vi "Lavatory_System..vi"(11 "Error_In":errorcluster) -> (15 "Error_Out":errorcluster)   [LabVIEW 2023]
doc: "This is the Main VI that performs the Lavatory system."
uses:
  Controls/Lavatory.ctl
  Controls/Lavatory_Data.ctl
  Controls/Queue_Operation_Select.ctl
  Controls/Timer_Operation_Select.ctl
panel:
  in  "Stop_Simulation":bool
  in  "Alarm_Timer_Limit":dbl=1.0 caption="Alarm Timer Limit" min=1.0 max=300.0
  out "Alarm_Timer_D":dbl caption="Alarm Timer D"
  out "Alarm_Timer_C":dbl caption="Alarm Timer C"
  in  "Lavatory_D_Occupied":bool caption="Lavatory D Occupied"
  in  "Lavatory_C_Occupied":bool caption="Lavatory C Occupied"
  out "Alarm_Timer_B":dbl caption="Alarm Timer B"
  out "Alarm_Timer_A":dbl caption="Alarm Timer A"
  in  "Lavatory_B_Occupied":bool caption="Lavatory B Occupied"
  in  "Lavatory_A_Occupied":bool caption="Lavatory A Occupied"
  out "Rear_Lavatories_Occupied":bool caption="Lavatories\nOccupied"
  out "Front_Lavatories_Occupied":bool caption="Lavatories\nOccupied"
  in  "Alarm_Achnowledge":bool caption="Alarm Achnowledge"
  out "Lavatory":string="Lavatory A,B,C,D"
  out "Alarm":bool
  in  "Seatbelt_Sign_ON":bool caption="Seatbelt Sign ON"
  out "Lavatory_A":T1 caption="Lavatory A"
  out "Lavatory_B":T1 caption="Lavatory B"
  out "Lavatory_D":T1 caption="Lavatory D"
  out "Lavatory_C":T1 caption="Lavatory C"
  # "Airplane Lavatory Signs"
  # "Front"
  # "Rear"
  # "Steward's Area"
  # "Simulation Contols & Indicators"
  # "Secs"
  # "Secs"
  # "Secs"
  # "Secs"
  # "Secs"
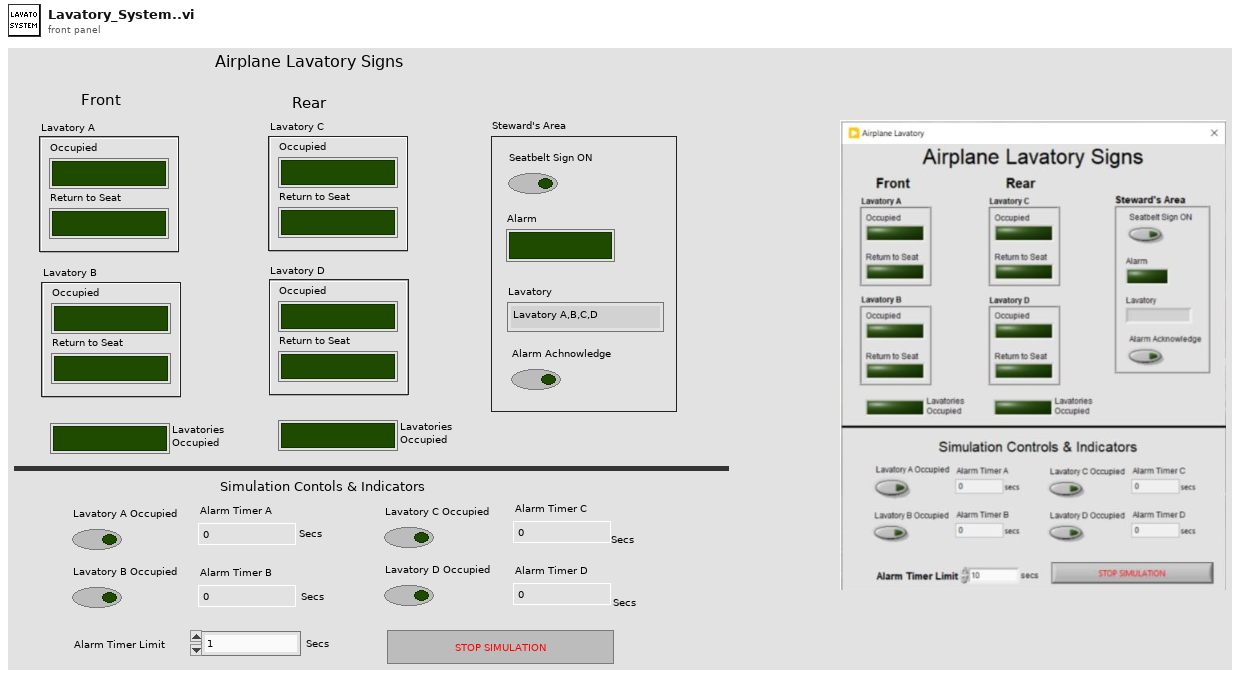
[diagram p1: front panel]
types:
  T1 = typedef "Lavatory.ctl" = cluster{"Occupied":bool, "Return_To_Seat":bool}
  T2 = typedef "Timer_Operation_Select.ctl" = enum16{"Initialize", "Start_Timer", "Time_Out?", "Stop_Timer"}
  T3 = typedef "Queue_Operation_Select.ctl" = enum16{"Obtain_Queue", "Enqueue", "Enqueue_N", "Enqueue_at_End", "Dequeue", "Flush", "Release_Queue"}
  T4 = typedef "Lavatory_Data.ctl" = cluster{"Lavatory":T1, "Rear_Lavatories_Occupied":bool, "Front_Lavatories_Occupied":bool, "Alarm_Time":dbl[], "Alarm":bool, "Alarm_Message":string, "Alarm_Timer_Limit":dbl, "Seatbelt_Sign_ON":bool, "Occupied":bool[], "Return_To_Seat_F":bool[], "Lavatory_Reference":refnum<vi>[], "Time_Out?":bool[], "Lavatory_Controls":refnum<vi>[]}
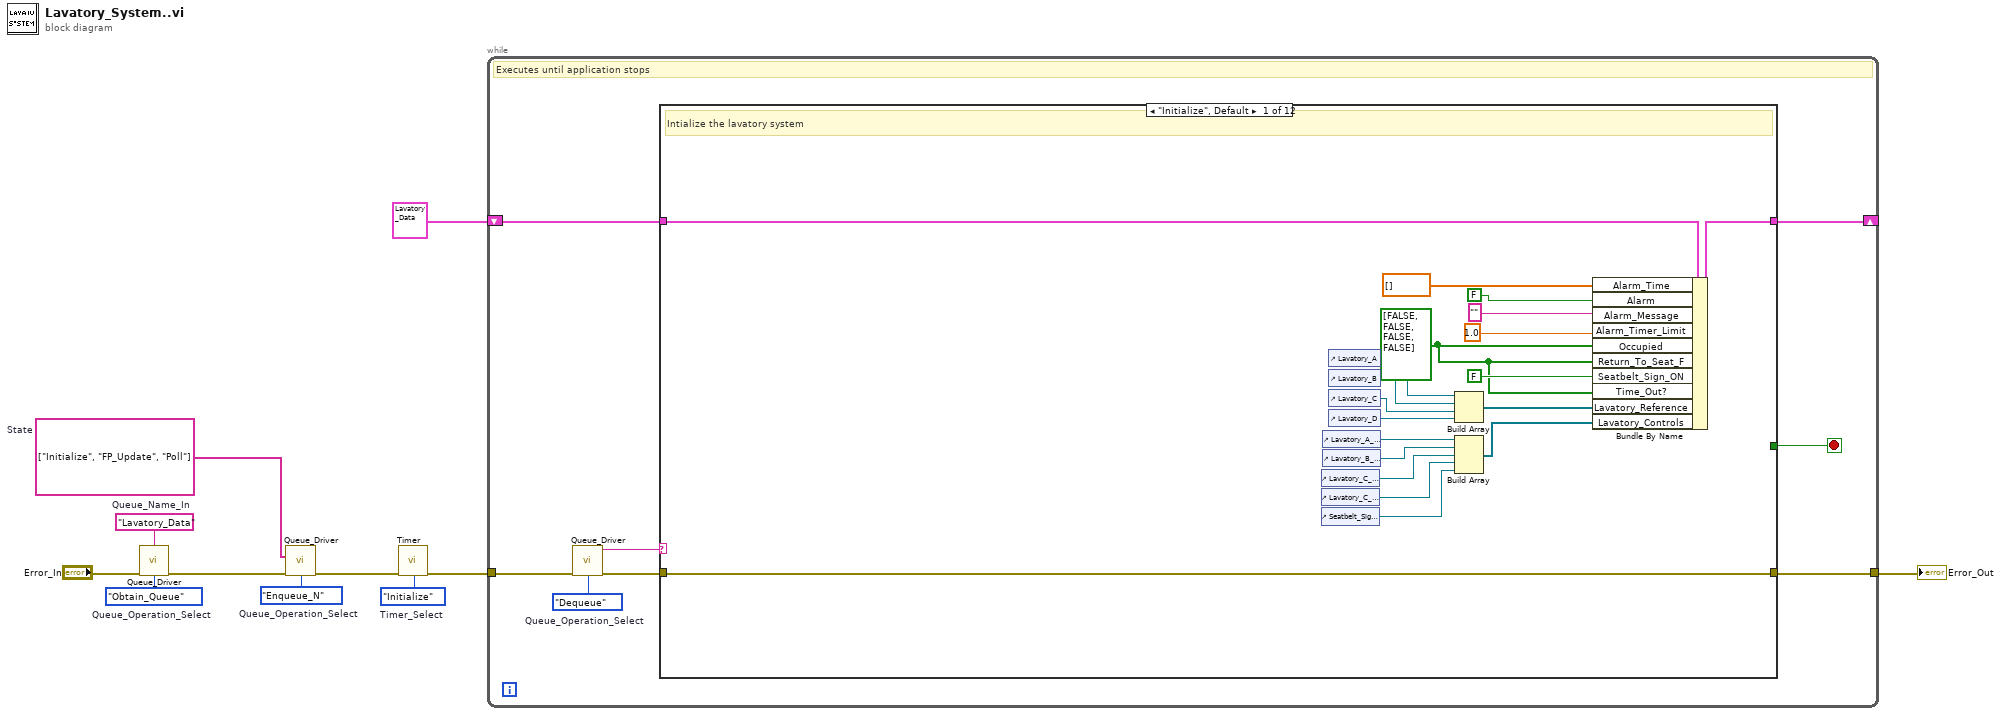
[diagram p0: block diagram]
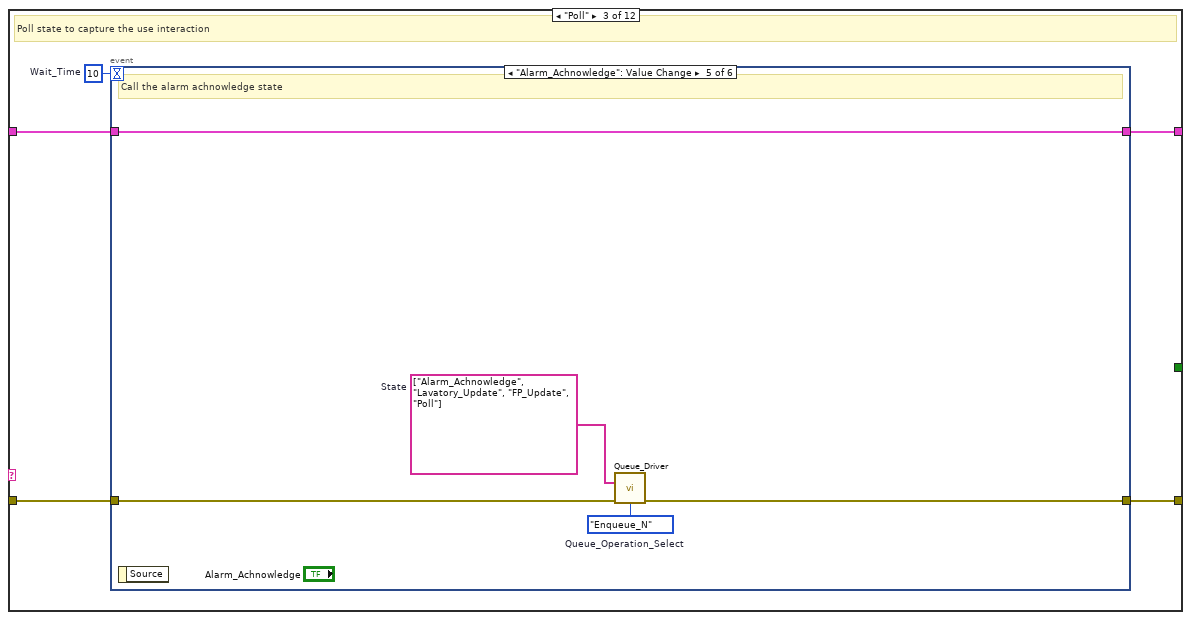
[diagram p3: hidden frame]
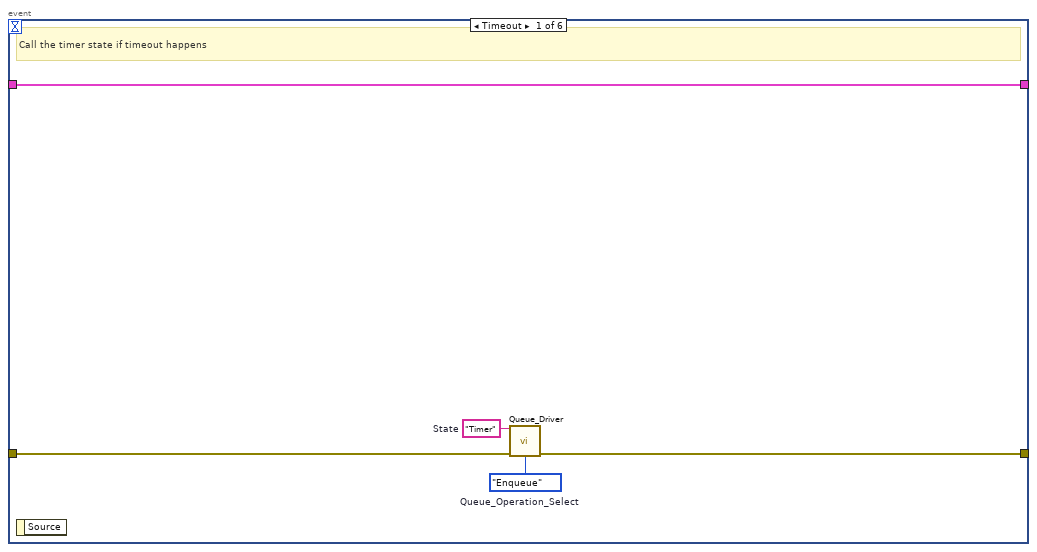
[diagram p4: hidden frame]
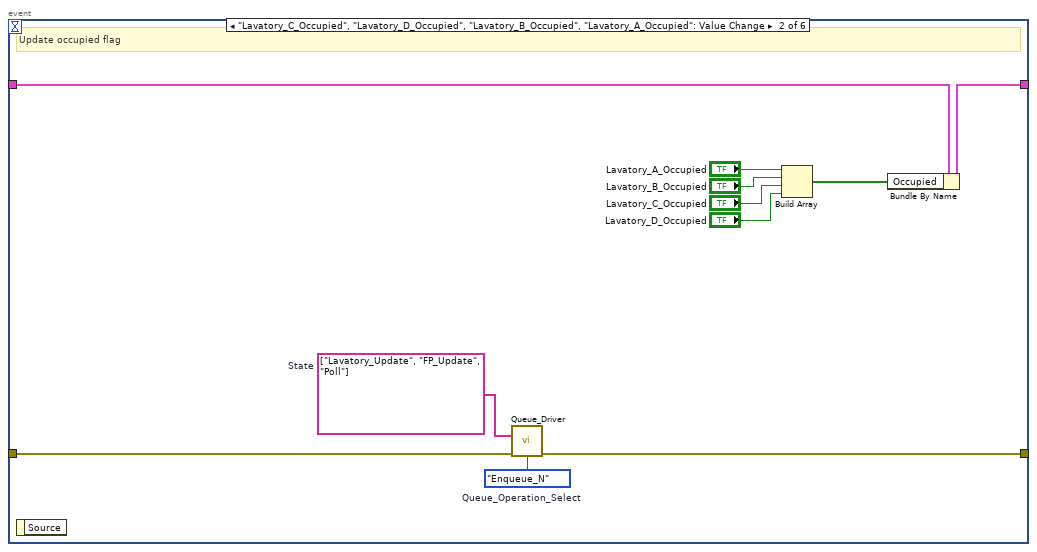
[diagram p5: hidden frame]
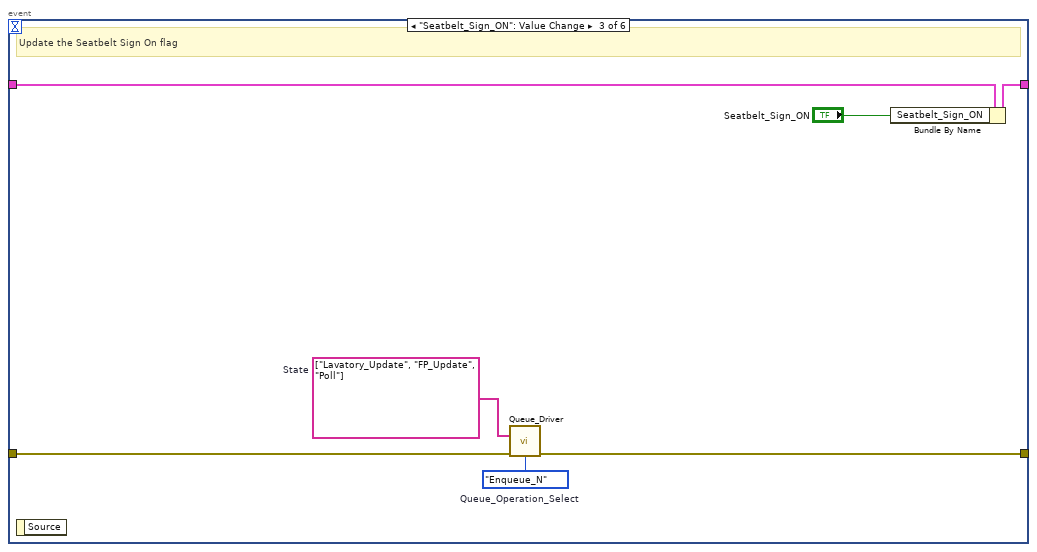
[diagram p6: hidden frame]
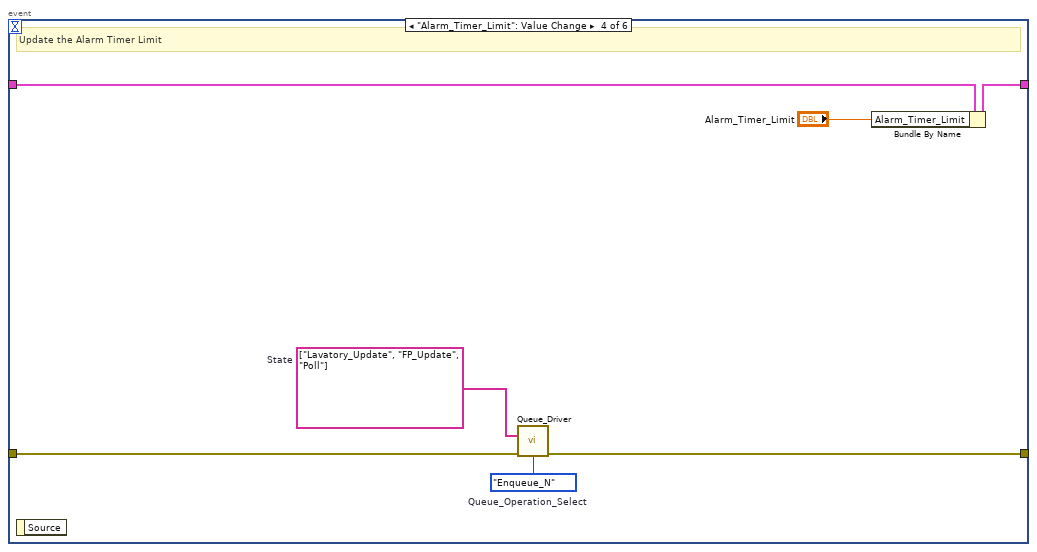
[diagram p7: hidden frame]
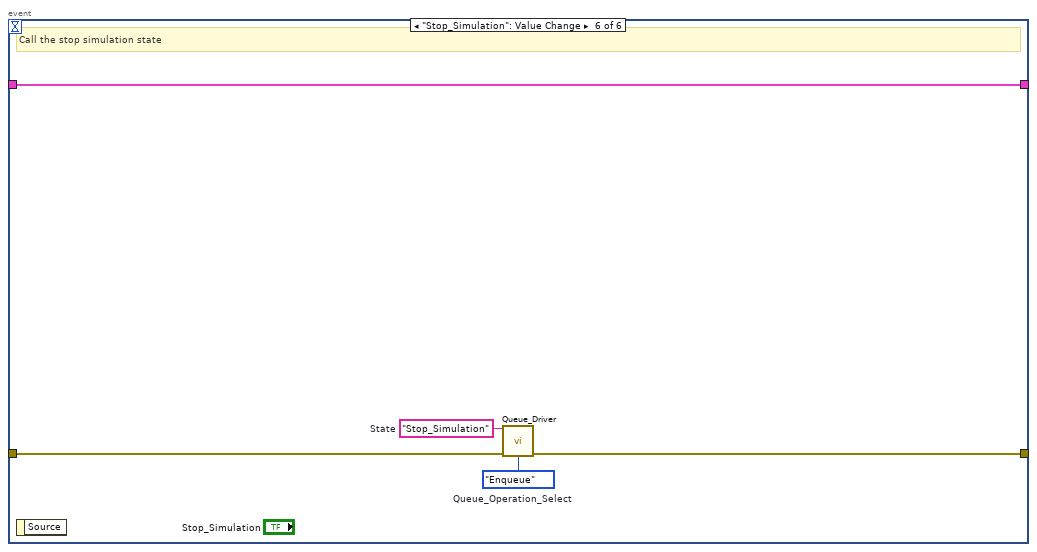
[diagram p8: hidden frame]
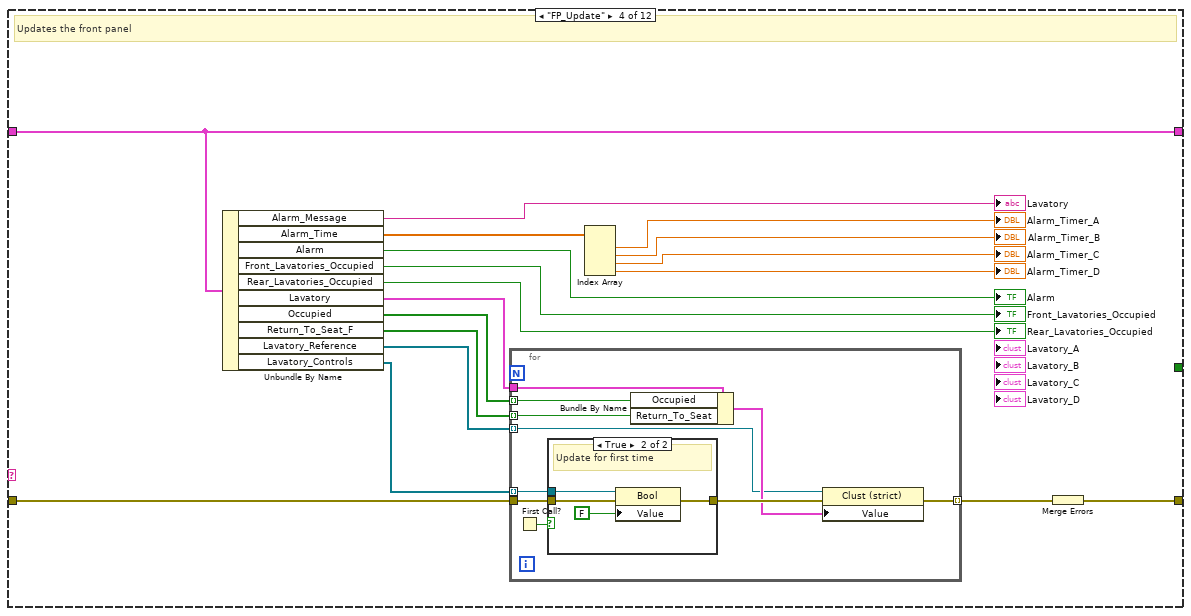
[diagram p9: hidden frame]
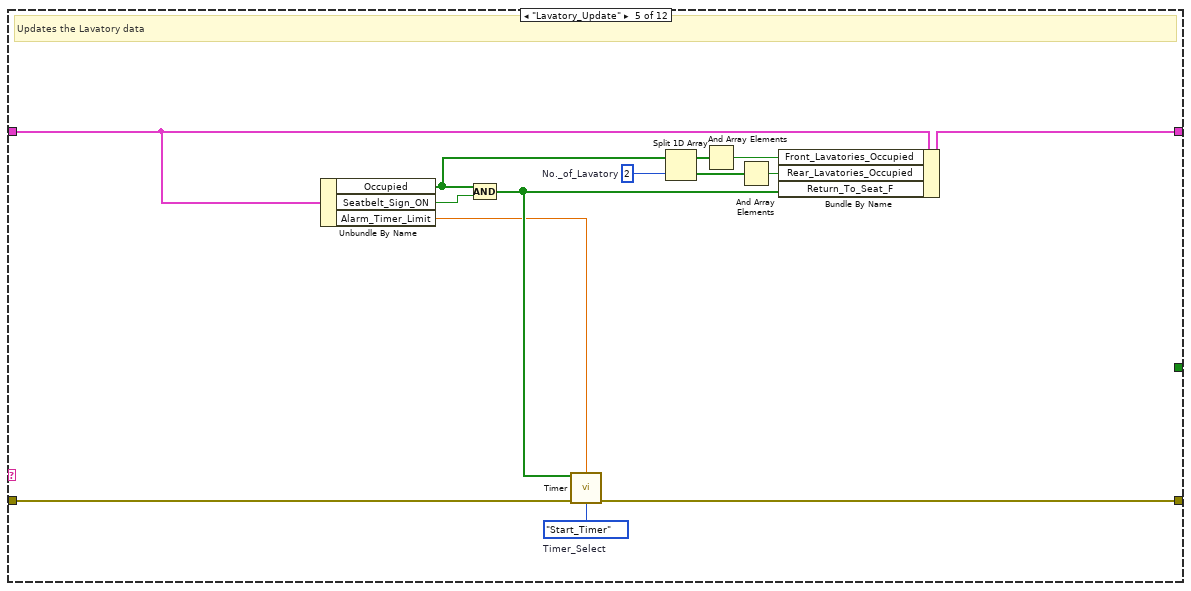
[diagram p11: hidden frame]
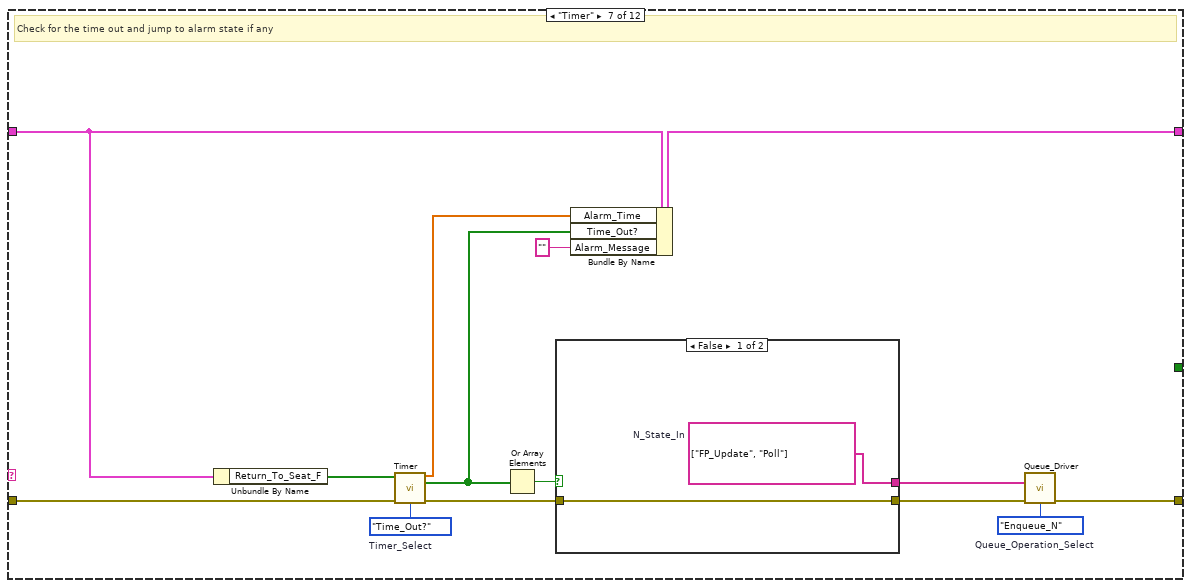
[diagram p13: hidden frame]
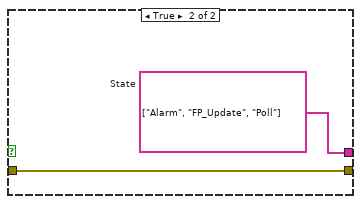
[diagram p14: hidden frame]
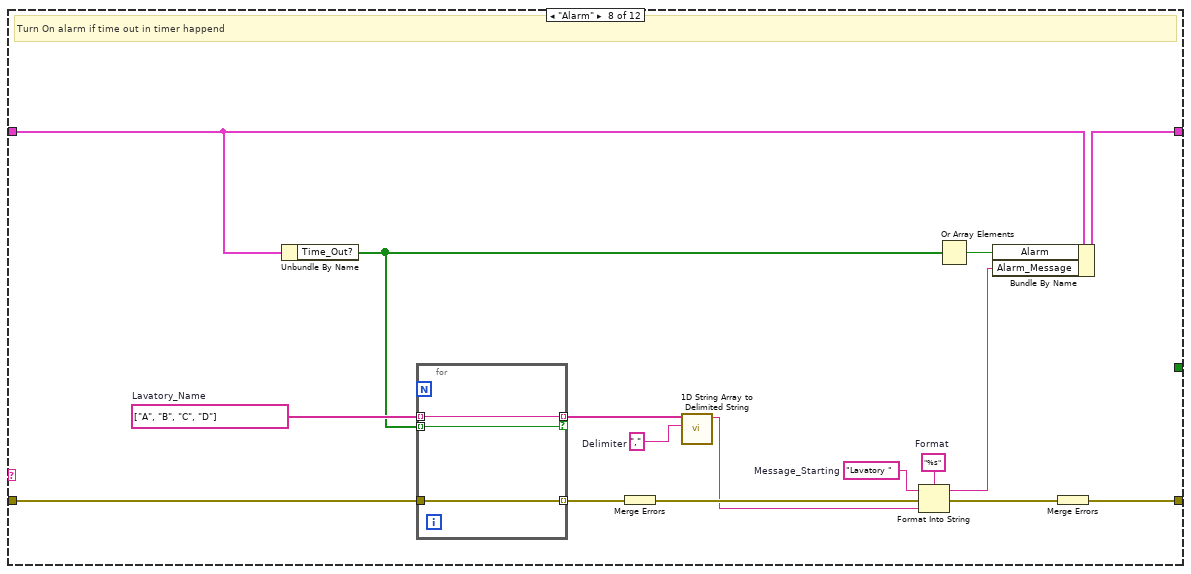
[diagram p15: hidden frame]
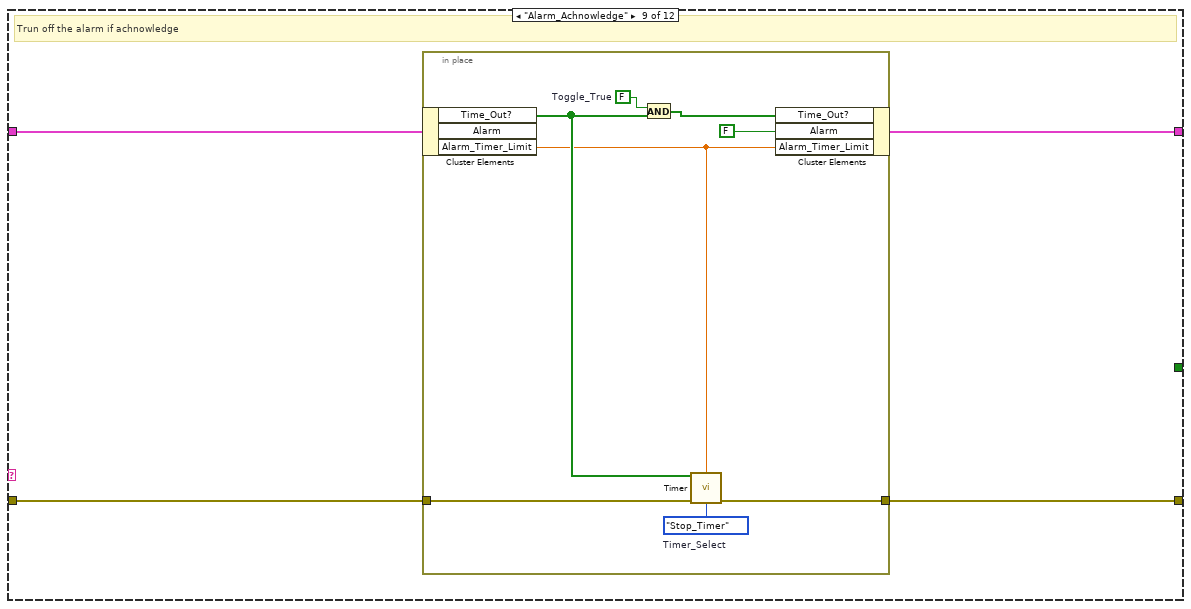
[diagram p16: hidden frame]
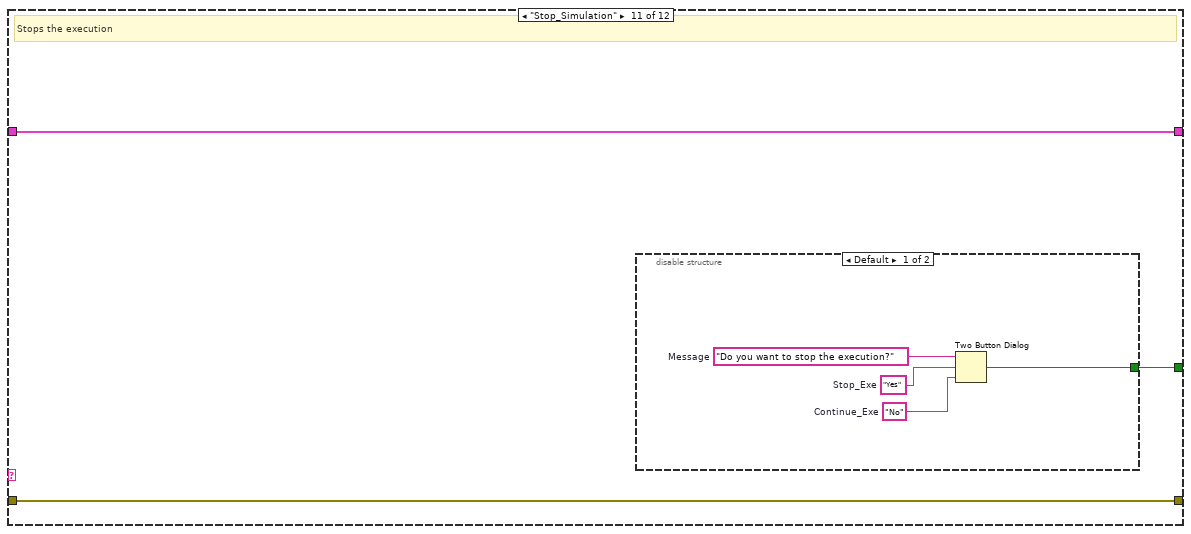
[diagram p18: hidden frame]
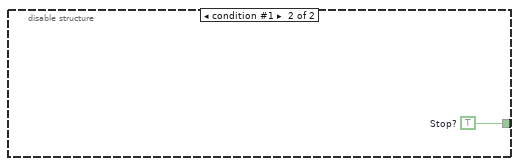
[diagram p19: hidden frame]
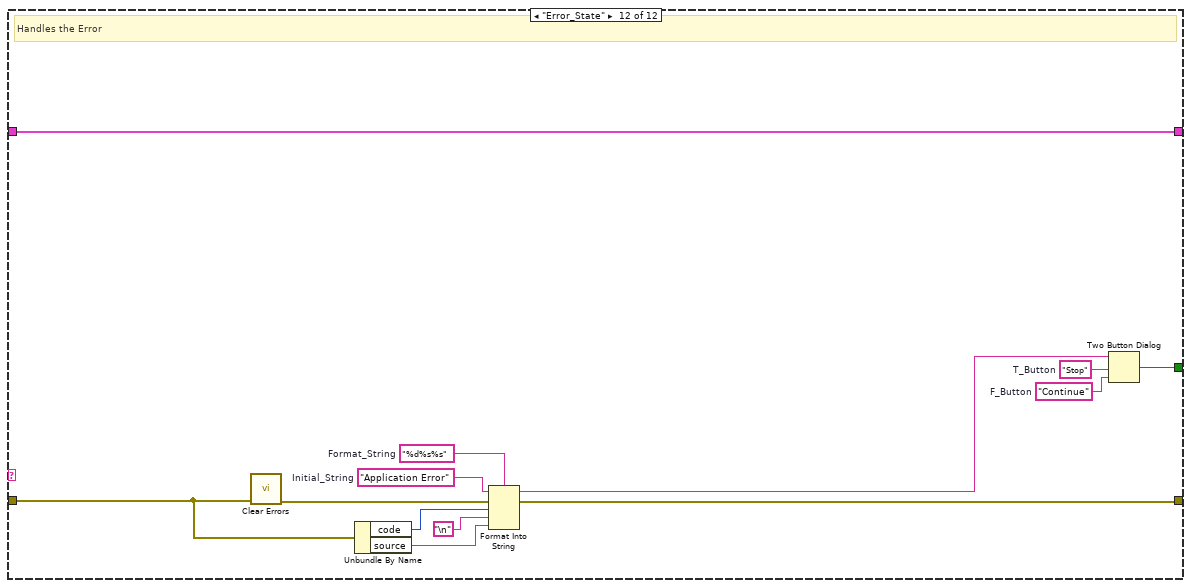
[diagram p20: hidden frame]
diagram:
  w1 = Timer_Operation_Select."Initialize"  # Timer_Select
  w4 = Queue_Operation_Select."Enqueue_N"  # Queue_Operation_Select
  w3 = string[] ["Initialize", "FP_Update", "Poll"]  # State
  w7 = Queue_Operation_Select."Obtain_Queue"  # Queue_Operation_Select
  w8 = "Lavatory_Data"  # Queue_Name_In
  n1 = call "Queue_Driver.vi"("Queue_Name_In"=w8, "Error_In"="Error_In", "Queue_Operation_Select"=w7) -> ("Error_Out"=w9:errorcluster)  [unwired: 11 in, 1 out]
  n2 = call "Queue_Driver.vi"("N_State_In"=w3, "Error_In"=w9, "Queue_Operation_Select"=w4) -> ("Error_Out"=w5:errorcluster)  [unwired: 11 in, 1 out]
  n3 = call "Timer.vi"("Error_In"=w5, "Timer_Select"=w1) -> ("Error_Out"=w2:errorcluster)  [unwired: 11 in, 2 out]
  n4 = while {
    tunnel: w2 -> [w18]
    tunnel: [w19] -> w10
    shift-right: [w14] -> _
    shift-left: T4 {"Lavatory"={"Occupied"=FALSE, "Return_To_Seat"=FALSE}, "Rear_Lavatories_Occupied"=FALSE, "Front_Lavatories_Occupied"=FALSE, "Alarm_Time"=[], "Alarm"=FALSE, "Alarm_Message"="", "Alarm_Timer_Limit"=0.0, "Seatbelt_Sign_ON"=FALSE, "Occupied"=[], "Return_To_Seat_F"=[], "Lavatory_Reference"=[], "Time_Out?"=[], "Lavatory_Controls"=[]} -> [w15]
    stop <- w12 stop-if-true
    w16 = Queue_Operation_Select."Dequeue"  # Queue_Operation_Select
    # "Executes until application stops"
    n5 = call "Queue_Driver.vi"("Error_In"=w18, "Queue_Operation_Select"=w16) -> ("State_Out"=w17:string, "Error_Out"=w13:errorcluster)  [unwired: 12 in]
    n6 = case shown="\"Initialize\", Default" w17 {
      tunnel: [w39 w40 w42 w94 w129 w134 w145 w167 w173 w185 w189 w197] -> w19
      tunnel: w13 -> [w39 w40 w46 w100 w133 w134 w148 w159 w174 w185 w189 w198]
      tunnel: w15 -> [w38 w41 w45 w101 w131 w135 w143 w169 w175 w186 w188 w195]
      tunnel: [w37 w41 w43 w101 w130 w135 w144 w166 w176 w186 w188 w195] -> w14
      tunnel: [_ _ _ _ _ _ _ _ _ _ w187 w196] -> w12
      frame "Initialize", Default {
        w30 = bool[] [FALSE, FALSE, FALSE, FALSE] ("Alarm_Achnowledge")
        # "Intialize the lavatory system"
        n7 = control-ref of="Lavatory_C_Occupied"() -> (w23:refnum<vi>)
        n8 = control-ref of="Lavatory_C_Occupied"() -> (w22:refnum<vi>)
        n9 = control-ref of="Seatbelt_Sign_ON"() -> (w20:refnum<vi>)
        n10 = control-ref of="Lavatory_A_Occupied"() -> (w25:refnum<vi>)
        n11 = control-ref of="Lavatory_B_Occupied"() -> (w24:refnum<vi>)
        n12 = control-ref of="Lavatory_A"() -> (w35:refnum<vi>)
        n13 = control-ref of="Lavatory_B"() -> (w34:refnum<vi>)
        n14 = control-ref of="Lavatory_C"() -> (w33:refnum<vi>)
        n15 = control-ref of="Lavatory_D"() -> (w32:refnum<vi>)
        n16 = Build Array(w35, w34, w33, w32) -> (w31:refnum<vi>[])
        n17 = Build Array(w25, w24, w23, w22, w20) -> (w21:refnum<vi>[])
        n18 = Bundle By Name(cluster=w38, "Alarm_Time"=dbl[] [] ("Alarm_Timer_A"), "Alarm"=FALSE ("Stop_Simulation"), "Alarm_Message"="" ("Lavatory"), "Alarm_Timer_Limit"=1.0, "Occupied"=w30, "Return_To_Seat_F"=w30, "Seatbelt_Sign_ON"=FALSE, "Time_Out?"=w30, "Lavatory_Reference"=w31, "Lavatory_Controls"=w21) -> (w37:T4)
      }
      frame "------------------Update_Users----------------" {
        # "States after this are caused due to user interaction"
      }
      frame "Poll" {
        w44 = 10  # Wait_Time
        # "Poll state to capture the use interaction"
        n19 = event shown="[4] \"Alarm_Achnowledge\": Value Change" {
          selector: _ -> [_ _ _ _ _ _]
          dyn-events: _ -> [_ _ _ _ _ _]
          timeout: w44 -> [_ _ _ _ _ _]
          tunnel: [w50 w59 w68 w72 w79 w84] -> w42
          tunnel: w46 -> [w51 w62 w69 w74 w80 w85]
          tunnel: w45 -> [w47 w61 w66 w76 w81 w86]
          tunnel: [w47 w60 w65 w75 w81 w86] -> w43
          event Timeout {
            w48 = "Timer"  # State
            w49 = Queue_Operation_Select."Enqueue"  # Queue_Operation_Select
            # "Call the timer state if timeout happens"
            n20 = event-data() -> ()  [unwired: 1 in, 1 out]
            n21 = call "Queue_Driver.vi"("State_In"=w48, "Error_In"=w51, "Queue_Operation_Select"=w49) -> ("Error_Out"=w50:errorcluster)  [unwired: 11 in, 1 out]
          }
          event "Lavatory_C_Occupied", "Lavatory_D_Occupied", "Lavatory_B_Occupied", "Lavatory_A_Occupied": Value Change {
            w57 = string[] ["Lavatory_Update", "FP_Update", "Poll"]  # State
            w58 = Queue_Operation_Select."Enqueue_N"  # Queue_Operation_Select
            # "Update occupied flag"
            n22 = event-data() -> ()  [unwired: 1 in, 1 out]
            n23 = call "Queue_Driver.vi"("N_State_In"=w57, "Error_In"=w62, "Queue_Operation_Select"=w58) -> ("Error_Out"=w59:errorcluster)  [unwired: 11 in, 1 out]
            n24 = Build Array("Lavatory_A_Occupied", "Lavatory_B_Occupied", "Lavatory_C_Occupied", "Lavatory_D_Occupied") -> (w52:bool[])
            n25 = Bundle By Name(cluster=w61, "Occupied"=w52) -> (w60:T4)
          }
          event "Seatbelt_Sign_ON": Value Change {
            w63 = string[] ["Lavatory_Update", "FP_Update", "Poll"]  # State
            w67 = Queue_Operation_Select."Enqueue_N"  # Queue_Operation_Select
            # "Update the Seatbelt Sign On flag"
            n26 = event-data() -> ()  [unwired: 1 in, 1 out]
            n27 = call "Queue_Driver.vi"("N_State_In"=w63, "Error_In"=w69, "Queue_Operation_Select"=w67) -> ("Error_Out"=w68:errorcluster)  [unwired: 11 in, 1 out]
            n28 = Bundle By Name(cluster=w66, "Seatbelt_Sign_ON"="Seatbelt_Sign_ON") -> (w65:T4)
          }
          event "Alarm_Timer_Limit": Value Change {
            w70 = string[] ["Lavatory_Update", "FP_Update", "Poll"]  # State
            w71 = Queue_Operation_Select."Enqueue_N"  # Queue_Operation_Select
            # "Update the Alarm Timer Limit"
            n29 = event-data() -> ()  [unwired: 1 in, 1 out]
            n30 = call "Queue_Driver.vi"("N_State_In"=w70, "Error_In"=w74, "Queue_Operation_Select"=w71) -> ("Error_Out"=w72:errorcluster)  [unwired: 11 in, 1 out]
            n31 = Bundle By Name(cluster=w76, "Alarm_Timer_Limit"="Alarm_Timer_Limit") -> (w75:T4)
          }
          event "Alarm_Achnowledge": Value Change {
            w77 = string[] ["Alarm_Achnowledge", "Lavatory_Update", "FP_Update", "Poll"]  # State
            w78 = Queue_Operation_Select."Enqueue_N"  # Queue_Operation_Select
            # "Call the alarm achnowledge state"
            n32 = event-data() -> ()  [unwired: 1 in, 1 out]
            n33 = call "Queue_Driver.vi"("N_State_In"=w77, "Error_In"=w80, "Queue_Operation_Select"=w78) -> ("Error_Out"=w79:errorcluster)  [unwired: 11 in, 1 out]
          }
          event "Stop_Simulation": Value Change {
            w82 = Queue_Operation_Select."Enqueue"  # Queue_Operation_Select
            w83 = "Stop_Simulation"  # State
            # "Call the stop simulation state"
            n34 = event-data() -> ()  [unwired: 1 in, 1 out]
            n35 = call "Queue_Driver.vi"("State_In"=w83, "Error_In"=w85, "Queue_Operation_Select"=w82) -> ("Error_Out"=w84:errorcluster)  [unwired: 11 in, 1 out]
          }
        }
      }
      frame "FP_Update" {
        # "Updates the front panel"
        n36 = Unbundle By Name(w101) -> ("Alarm_Message"=→"Lavatory":string, "Alarm_Time"=w92:dbl[], "Alarm"=→"Alarm":bool, "Front_Lavatories_Occupied"=→"Front_Lavatories_Occupied":bool, "Rear_Lavatories_Occupied"=→"Rear_Lavatories_Occupied":bool, "Lavatory"=w96:T1, "Occupied"=w98:bool[], "Return_To_Seat_F"=w97:bool[], "Lavatory_Reference"=w95:refnum<vi>[], "Lavatory_Controls"=w87:refnum<vi>[])
        n37 = for {
          tunnel: w95 -> [w105] mode=indexing
          tunnel: w98 -> [w111] mode=indexing
          tunnel: w97 -> [w112] mode=indexing
          tunnel: w96 -> [w107]
          tunnel: w100 -> [w114]
          tunnel: [w113] -> w99 mode=indexing
          tunnel: w87 -> [w109] mode=indexing
          n38 = First Call?() -> (First Call?: T/F=w108:bool)
          n39 = case shown="True" w108 {
            tunnel: w114 -> [w115 w119]
            tunnel: [w115 w118] -> w110
            tunnel: w109 -> [_ w117]
            frame False {
            }
            frame True {
              # "Update for first time"
              n40 = property on="Property Node" class="Bool"(reference=w117, error in=w119, "Value"=FALSE) -> (error out=w118:errorcluster)  [unwired: 1 out]
            }
          }
          n41 = Bundle By Name(cluster=w107, "Occupied"=w111, "Return_To_Seat"=w112) -> (w106:T1)
          n42 = property on="Property Node" class="Clust (strict)"(reference=w105, error in=w110, "Value"=w106) -> (error out=w113:errorcluster)  [unwired: 1 out]
        }
        n43 = Index Array(array=w92) -> (element #1=→"Alarm_Timer_A":dbl, element #2=→"Alarm_Timer_B":dbl, element #3=→"Alarm_Timer_C":dbl, element #4=→"Alarm_Timer_D":dbl)  [unwired: 4 in]
        n44 = Merge Errors(w99) -> (w94:errorcluster)
      }
      frame "Lavatory_Update" {
        w123 = 2  # No._of_Lavatory
        w132 = Timer_Operation_Select."Start_Timer"  # Timer_Select
        # "Updates the Lavatory data"
        n45 = Unbundle By Name(w131) -> ("Occupied"=w121:bool[], "Seatbelt_Sign_ON"=w122:bool, "Alarm_Timer_Limit"=w120:dbl)
        n46 = Compound Arithmetic op=AND(w121, w122) -> (w128:bool[])
        n47 = call "Timer.vi"("Timers_Start"=w128, "Wait_Time"=w120, "Error_In"=w133, "Timer_Select"=w132) -> ("Error_Out"=w129:errorcluster)  [unwired: 9 in, 2 out]
        n48 = Split 1D Array(array=w121, index=w123) -> (first subarray=w127:bool[], second subarray=w125:bool[])
        n49 = And Array Elements(Boolean array=w127) -> (logical AND=w126:bool)
        n50 = And Array Elements(Boolean array=w125) -> (logical AND=w124:bool)
        n51 = Bundle By Name(cluster=w131, "Front_Lavatories_Occupied"=w126, "Rear_Lavatories_Occupied"=w124, "Return_To_Seat_F"=w128) -> (w130:T4)
      }
      frame "-----------------Timer_and_Alarm-------------" {
        # "States after this are timer and alarm related states"
      }
      frame "Timer" {
        w146 = Queue_Operation_Select."Enqueue_N"  # Queue_Operation_Select
        w149 = Timer_Operation_Select."Time_Out?"  # Timer_Select
        # "Check for the time out and jump to alarm state if any"
        n52 = Unbundle By Name(w143) -> ("Return_To_Seat_F"=w142:bool[])
        n53 = call "Timer.vi"("Timers_Start"=w142, "Error_In"=w148, "Timer_Select"=w149) -> ("Timer_Time"=w140:dbl[], "Time_Out?"=w136:bool[], "Error_Out"=w138:errorcluster)  [unwired: 10 in]
        n54 = Or Array Elements(Boolean array=w136) -> (logical OR=w137:bool)
        n55 = case shown="False" w137 {
          tunnel: [w150 w153] -> w147
          tunnel: [w151 w152] -> w139
          tunnel: w138 -> [w151 w152]
          frame False {
            w150 = string[] ["FP_Update", "Poll"]  # N_State_In
          }
          frame True {
            w153 = string[] ["Alarm", "FP_Update", "Poll"]  # State
          }
        }
        n56 = Bundle By Name(cluster=w143, "Alarm_Time"=w140, "Time_Out?"=w136, "Alarm_Message"="" ("Lavatory")) -> (w144:T4)
        n57 = call "Queue_Driver.vi"("N_State_In"=w147, "Error_In"=w139, "Queue_Operation_Select"=w146) -> ("Error_Out"=w145:errorcluster)  [unwired: 11 in, 1 out]
      }
      frame "Alarm" {
        w155 = ","  # Delimiter
        w163 = "%s"  # Format
        w168 = string[] ["A", "B", "C", "D"]  # Lavatory_Name
        w162 = "Lavatory "  # Message_Starting
        # "Turn On alarm if time out in timer happend"
        n58 = Unbundle By Name(w169) -> ("Time_Out?"=w164:bool[])
        n59 = for {
          tunnel: w164 -> [w170] mode=indexing
          tunnel: w168 -> [w171] mode=indexing
          tunnel: w159 -> [w172]
          tunnel: [w172] -> w158 mode=indexing
          tunnel: [w171] -> w156 mode=indexing if=w170
        }
        n60 = Merge Errors(w158) -> (w157:errorcluster)
        n61 = call <vilib>:"1D String Array to Delimited String.vi"("delimiter"=w155, "string array"=w156) -> ("delimited string"=w154:string)  [unwired: 9 in]
        n62 = Format Into String(format string=w163, initial string=w162, error in=w157, w154) -> (resulting string=w161:string, error out=w160:errorcluster)
        n63 = Or Array Elements(Boolean array=w164) -> (logical OR=w165:bool)
        n64 = Bundle By Name(cluster=w169, "Alarm"=w165, "Alarm_Message"=w161) -> (w166:T4)
        n65 = Merge Errors(w160) -> (w167:errorcluster)
      }
      frame "Alarm_Achnowledge" {
        # "Trun off the alarm if achnowledge"
        n66 = in-place "In Place Element Structure" {
          in-place-border: w174 -> [w184]
          in-place-border: [w183] -> w173
          w182 = Timer_Operation_Select."Stop_Timer"  # Timer_Select
          w179 = FALSE  # Toggle_True
          n67 = in-place-cluster #1(w175) -> ("Time_Out?"=w178:bool[], "Alarm_Timer_Limit"=w177:dbl)  [unwired: 1 out]
          n68 = And(x=w179, y=w178) -> (x .and. y?=w180:bool[])
          n69 = call "Timer.vi"("Timers_Start"=w178, "Wait_Time"=w177, "Error_In"=w184, "Timer_Select"=w182) -> ("Error_Out"=w183:errorcluster)  [unwired: 9 in, 2 out]
          n70 = in-place-cluster #1("Time_Out?"=w180, "Alarm"=FALSE, "Alarm_Timer_Limit"=w177) -> (w176:T4)
        }
      }
      frame "----------------------- Exit---------------------" {
        # "States after this are exit related"
      }
      frame "Stop_Simulation" {
        # "Stops the execution"
        n71 = disable-structure "Conditional Disable Structure" shown="Default" {
          disable-tunnel: [w190 w194] -> w187
          frame condition #0 (active) {
            w191 = "No"  # Continue_Exe
            w192 = "Yes"  # Stop_Exe
            w193 = "Do you want to stop the execution?"  # Message
            n72 = Two Button Dialog(message=w193, 1:w191, 2:w192) -> (T button?=w190:bool)
          }
          frame condition #1 {
            w194 = TRUE  # Stop?
          }
        }
      }
      frame "Error_State" {
        w203 = "%d%s%s"  # Format_String
        w204 = "Application Error"  # Initial_String
        w205 = "Stop"  # T_Button
        w206 = "Continue"  # F_Button
        # "Handles the Error"
        n73 = call <vilib>:"Clear Errors.vi"("error in (no error)"=w198) -> ("error out"=w201:errorcluster)  [unwired: 5 in, 1 out]
        n74 = Unbundle By Name(w198) -> ("code"=w200:i32, "source"=w199:string)
        n75 = Format Into String(format string=w203, initial string=w204, error in=w201, w200, "\n" ("Line Feed Constant"), w199) -> (resulting string=w207:string, error out=w197:errorcluster)
        n76 = Two Button Dialog(message=w207, 1:w206, 2:w205) -> (T button?=w196:bool)
      }
    }
  }
  "Error_Out" <- w10
